vi "电源管理UI.vi"() -> ()   [LabVIEW 2016, in "PLC.lvlib"]
uses:
  PLC.lvlib
  <vilib>/Utility/miscctls.llb/LVPointTypeDef.ctl
panel:
  in  "CODCr电源":bool
  in  "总磷总氮电源":bool
  in  "营养盐电源":bool
  in  "CODMn电源":bool
  in  "多参数电源":bool
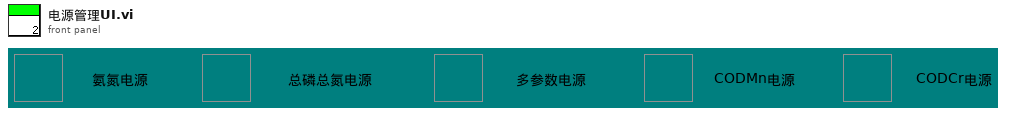
[diagram p1: front panel]
types:
  T1 = typedef "LVPointTypeDef.ctl" = cluster{"Horizontal":i16, "Vertical":i16}
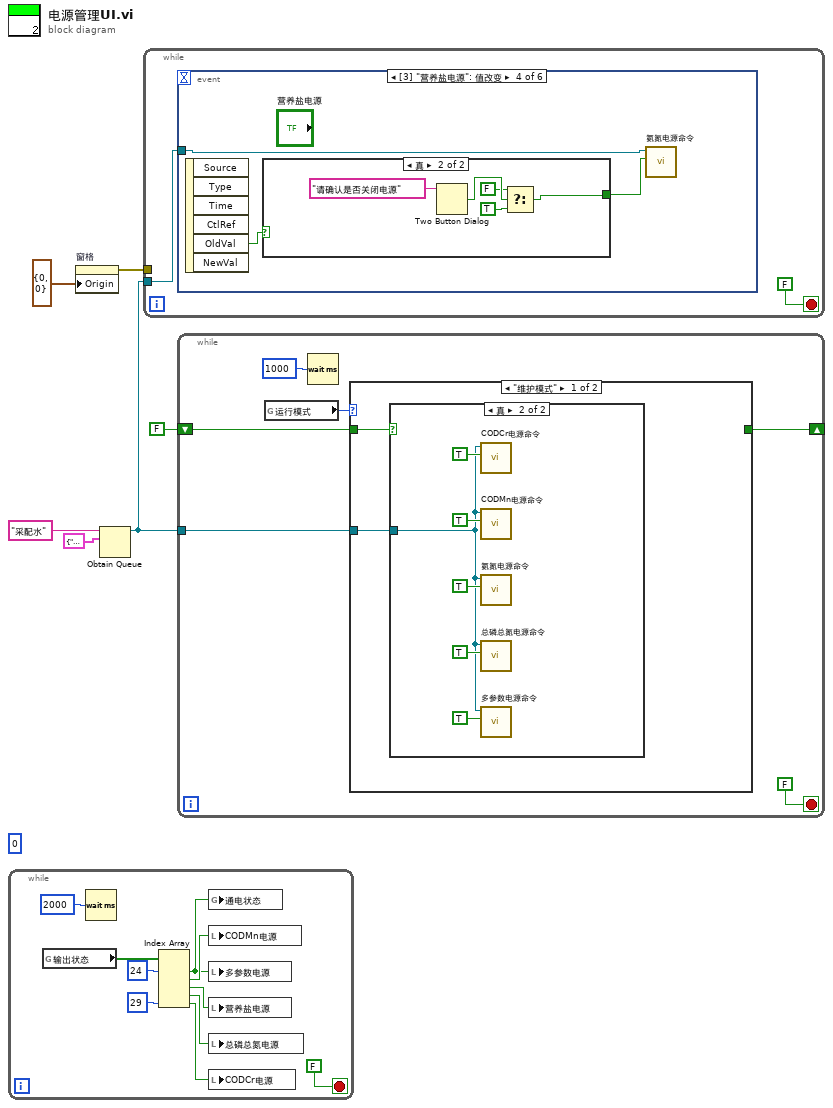
[diagram p0: block diagram]
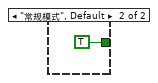
[diagram p3: hidden frame]
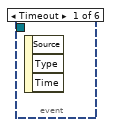
[diagram p4: hidden frame]
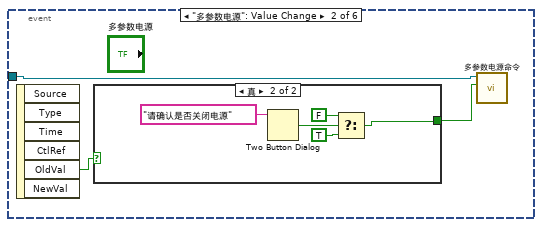
[diagram p5: hidden frame]
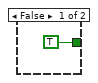
[diagram p6: hidden frame]
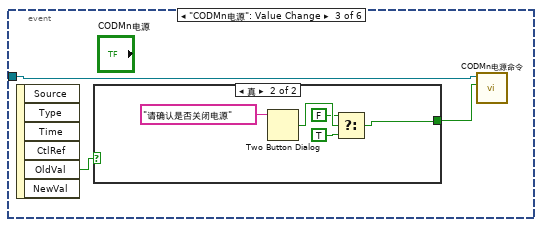
[diagram p7: hidden frame]
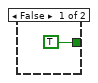
[diagram p8: hidden frame]
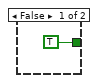
[diagram p9: hidden frame]
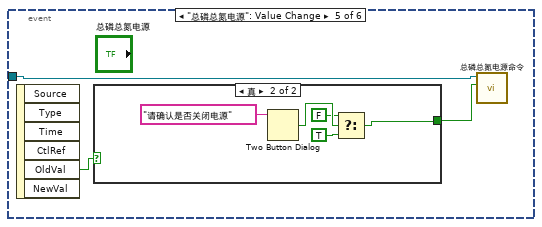
[diagram p10: hidden frame]
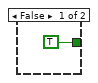
[diagram p11: hidden frame]
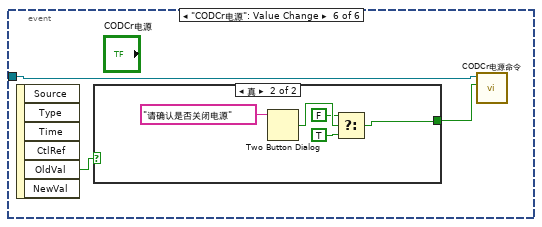
[diagram p12: hidden frame]
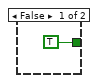
[diagram p13: hidden frame]
diagram:
  (unwired) u32 0 ("等待时间（毫秒）")
  n1 = while {
    stop <- FALSE stop-if-true
    n2 = global read "采配水全局变量.vi" "输出状态"() -> (w14:bool[])
    n3 = Wait (ms)(milliseconds to wait=u32 2000 ("等待时间（毫秒）")) -> ()  [unwired: 1 out]
    n4 = Index Array(array=w14, index #1=24 ("索引"), index #5=29 ("索引")) -> (element #1=w9:bool, element #2=w12:bool, element #3=w11:bool, element #4=w10:bool, element #5=w8:bool)  [unwired: 3 in]
    n5 = global write "多参数全局变量.vi" "通电状态"(w9) -> ()
    n6 = local write "CODMn电源"(w12) -> ()
    n7 = local write "多参数电源"(w9) -> ()
    n8 = local write "营养盐电源"(w11) -> ()
    n9 = local write "总磷总氮电源"(w10) -> ()
    n10 = local write "CODCr电源"(w8) -> ()
  }
  n11 = property on="窗格" class="Pane"("Origin"=T1 {"Horizontal"=0, "Vertical"=0} ("原点")) -> (error out=w3:errorcluster)  [unwired: 2 in, 1 out]
  n12 = Obtain Queue(name (unnamed)="采配水" ("名称（未命名）"), element data type=cluster{"命令":string, "数据":variant} {"命令"="", "数据"=variant}) -> (queue out=w2:refnum<queue>)  [unwired: 3 in, 2 out]
  n13 = while {
    tunnel: w2 -> [w17]
    tunnel: w3 -> [_]
    stop <- FALSE stop-if-true
    n14 = event shown="[3] \"营养盐电源\": 值改变" {
      selector: _ -> [_ _ _ _ _ _]
      dyn-events: _ -> [_ _ _ _ _ _]
      timeout: _ -> [_ _ _ _ _ _]
      tunnel: w17 -> [_ w21 w30 w39 w48 w57]
      event Timeout {
        n15 = event-data() -> ()  [unwired: 1 in, 3 out]
      }
      event "多参数电源": Value Change {
        n16 = event-data() -> ("OldVal"=w20:bool)  [unwired: 1 in, 5 out]
        n17 = case shown="真" w20 {
          tunnel: [TRUE ("T button?") w23] -> w19
          frame False {
          }
          frame True {
            n18 = Two Button Dialog(message="请确认是否关闭电源" ("消息")) -> (T button?=w26:bool)  [unwired: 2 in]
            n19 = Select(t=FALSE, s=w26, f=TRUE ("T button?")) -> (s? t:f=w23:bool)
          }
        }
        n20 = call "多参数电源命令.vi"("通电/断电"=w19, "队列"=w21) -> ()  [unwired: 9 in, 1 out]
      }
      event "CODMn电源": Value Change {
        n21 = event-data() -> ("OldVal"=w29:bool)  [unwired: 1 in, 5 out]
        n22 = case shown="真" w29 {
          tunnel: [TRUE ("T button?") w32] -> w28
          frame False {
          }
          frame True {
            n23 = Two Button Dialog(message="请确认是否关闭电源" ("消息")) -> (T button?=w35:bool)  [unwired: 2 in]
            n24 = Select(t=FALSE, s=w35, f=TRUE ("T button?")) -> (s? t:f=w32:bool)
          }
        }
        n25 = call "CODMn电源命令.vi"("通电/断电"=w28, "队列"=w30) -> ()  [unwired: 9 in, 1 out]
      }
      event "营养盐电源": Value Change {
        n26 = event-data() -> ("OldVal"=w38:bool)  [unwired: 1 in, 5 out]
        n27 = case shown="真" w38 {
          tunnel: [TRUE ("T button?") w41] -> w37
          frame False {
          }
          frame True {
            n28 = Two Button Dialog(message="请确认是否关闭电源" ("消息")) -> (T button?=w44:bool)  [unwired: 2 in]
            n29 = Select(t=FALSE, s=w44, f=TRUE ("T button?")) -> (s? t:f=w41:bool)
          }
        }
        n30 = call "氨氮电源命令.vi"("通电/断电"=w37, "队列"=w39) -> ()  [unwired: 9 in, 1 out]
      }
      event "总磷总氮电源": Value Change {
        n31 = event-data() -> ("OldVal"=w47:bool)  [unwired: 1 in, 5 out]
        n32 = case shown="真" w47 {
          tunnel: [TRUE ("T button?") w50] -> w46
          frame False {
          }
          frame True {
            n33 = Two Button Dialog(message="请确认是否关闭电源" ("消息")) -> (T button?=w53:bool)  [unwired: 2 in]
            n34 = Select(t=FALSE, s=w53, f=TRUE ("T button?")) -> (s? t:f=w50:bool)
          }
        }
        n35 = call "总磷总氮电源命令.vi"("通电/断电"=w46, "队列"=w48) -> ()  [unwired: 9 in, 1 out]
      }
      event "CODCr电源": Value Change {
        n36 = event-data() -> ("OldVal"=w56:bool)  [unwired: 1 in, 5 out]
        n37 = case shown="真" w56 {
          tunnel: [TRUE ("T button?") w59] -> w55
          frame False {
          }
          frame True {
            n38 = Two Button Dialog(message="请确认是否关闭电源" ("消息")) -> (T button?=w62:bool)  [unwired: 2 in]
            n39 = Select(t=FALSE, s=w62, f=TRUE ("T button?")) -> (s? t:f=w59:bool)
          }
        }
        n40 = call "CODCr电源命令.vi"("通电/断电"=w55, "队列"=w57) -> ()  [unwired: 9 in, 1 out]
      }
    }
  }
  n41 = while {
    tunnel: w2 -> [w67]
    shift-right: [w64] -> _
    shift-left: FALSE -> [w65]
    stop <- FALSE stop-if-true
    n42 = global read "系统设置全局变量.vi" "运行模式"() -> (w66:enum16{"维护模式", "常规模式", "应急模式", "质控模式"})
    n43 = Wait (ms)(milliseconds to wait=u32 1000 ("等待时间（毫秒）")) -> ()  [unwired: 1 out]
    n44 = case shown="\"维护模式\"" w66 {
      tunnel: w67 -> [w71 _]
      tunnel: w65 -> [w70 _]
      tunnel: [_ TRUE] -> w64
      frame "维护模式" {
        n45 = case shown="真" w70 {
          tunnel: w71 -> [_ w72]
          frame False {
          }
          frame True {
            n46 = call "CODCr电源命令.vi"("通电/断电"=TRUE, "队列"=w72) -> ()  [unwired: 9 in, 1 out]
            n47 = call "CODMn电源命令.vi"("通电/断电"=TRUE, "队列"=w72) -> ()  [unwired: 9 in, 1 out]
            n48 = call "氨氮电源命令.vi"("通电/断电"=TRUE, "队列"=w72) -> ()  [unwired: 9 in, 1 out]
            n49 = call "总磷总氮电源命令.vi"("通电/断电"=TRUE, "队列"=w72) -> ()  [unwired: 9 in, 1 out]
            n50 = call "多参数电源命令.vi"("通电/断电"=TRUE, "队列"=w72) -> ()  [unwired: 9 in, 1 out]
          }
        }
      }
      frame "常规模式", Default {
      }
    }
  }
